vi "Day2.vi"   [LabVIEW 2019]
uses:
  <vilib>/Utility/file.llb/Read Delimited Spreadsheet (I64).vi
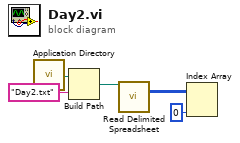
[diagram p0: block diagram]
diagram:
  n1 = call <vilib>:"Application Directory.vi"() -> ("Application Directory"=w5:path)
  n2 = Build Path(base path=w5, name or relative path="Day2.txt") -> (appended path=w3:path)
  n3 = call-poly <vilib>:"Read Delimited Spreadsheet.vi"("file path (dialog if empty)"=w3) -> ("all rows"=w2:i64[][])  [unwired: 9 in, 5 out]
  n4 = Index Array(array=w2, index (col)=0 ("disabled index (col)")) -> ()  [unwired: 1 in, 1 out]
